vi "list_word_docs.vi"(8 "error in (no error)":errorcluster) -> (0 "error out":errorcluster, 2 "DocumentNames":string[](array[string]), 3 "DocumentPaths":string[](array[string]))   [LabVIEW 2018]
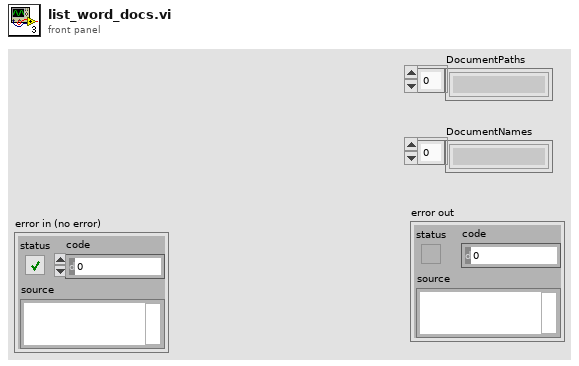
[diagram p1: front panel]
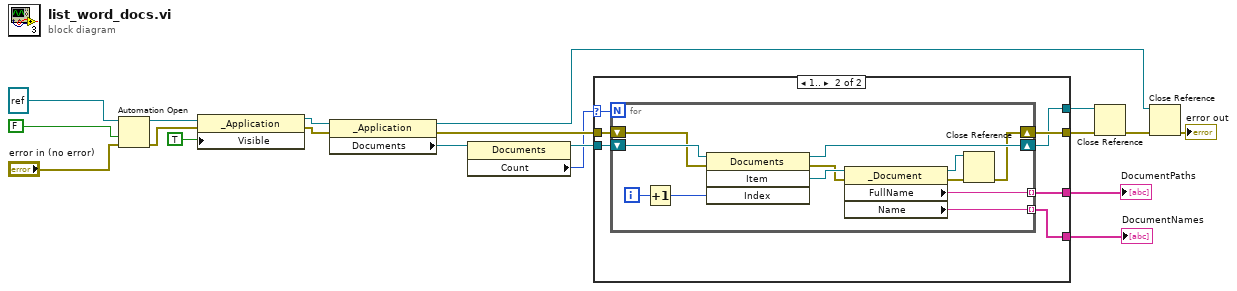
[diagram p0: block diagram]
diagram:
  n1 = Automation Open(error in (no error)="error in (no error)", Automation Refnum=refnum<k7> refnum ("Word._Application"), 9:FALSE ("open new instance (false)")) -> (Automation Refnum=w17:refnum<k7>, error out=w15:errorcluster)  [unwired: 1 in]
  n2 = property class="_Application"(reference=w17, error in=w15, "Visible"=TRUE) -> (reference out=w14:refnum<k7>, error out=w13:errorcluster)
  n3 = property class="_Application"(reference=w14, error in=w13) -> (reference out=w8:refnum<k7>, error out=w12:errorcluster, "Documents"=w5:refnum<k7>)
  n4 = property class="Documents"(reference=w5) -> (reference out=w4:refnum<k7>, "Count"=w1:i32)  [unwired: 1 in, 1 out]
  n5 = case shown="1.." w1 {
    selector: w1 -> [_ w22]
    tunnel: w12 -> [w20 w28]
    tunnel: [w20 w27] -> w10
    tunnel: [_ w26] -> w6
    tunnel: w4 -> [w21 w25]
    tunnel: [_ w24] -> w3
    tunnel: [w21 w23] -> w2
    frame ..0 {
    }
    frame 1.. {
      n6 = for {
        N: w22 -> [_]
        shift-right: [w30] -> w27
        shift-left: w28 -> [w38]
        shift-right: [w34] -> w23
        shift-left: w25 -> [w39]
        tunnel: [w40] -> w26 mode=indexing
        tunnel: [w29] -> w24 mode=indexing
        i -> [w37]
        n7 = Increment(x=w37) -> (x+1=w36:i32)
        n8 = invoke class="Documents" method="Item"(reference=w39, error in=w38, "Index"=w36) -> (reference out=w34:refnum<k7>, error out=w31:errorcluster, "Item"=w35:refnum<k7>)  [unwired: 1 in, 1 out]
        n9 = property class="_Document"(reference=w35, error in=w31) -> (reference out=w33:refnum<k7>, error out=w32:errorcluster, "FullName"=w40:string, "Name"=w29:string)
        n10 = Close Reference(reference=w33, error in (no error)=w32) -> (error out=w30:errorcluster)
      }
    }
  }
  "DocumentPaths" <- w6
  "DocumentNames" <- w3
  n11 = Close Reference(reference=w2, error in (no error)=w10) -> (error out=w7:errorcluster)
  n12 = Close Reference(reference=w8, error in (no error)=w7) -> (error out=→"error out":errorcluster)
